vi "Run.vi"(8 "error in (no error)":errorcluster caption="entrée d'erreur (pas d'erreur)", 9 "Y":string[][](array[string]), 10 "X":string[][](array[string]), 11 "Pairwise_distances.lvclass":refnum<class "Pairwise_distances.lvclass">) -> (0 "error out":errorcluster caption="sortie d'erreur", 2 "Data":T1, 3 "Pairwise_distances.lvclass":refnum<class "Pairwise_distances.lvclass">)   [LabVIEW 2020, in "Pairwise_distances.lvclass"]
doc: "Returns : \n\n- D : array [n_samples_a, n_samples_a] or [n_samples_a, n_samples_b]\nA distance matrix D such that D_{i, j} is the distance between the ith and jth vectors of the given matrix X, if Y is None. If Y is not None, then D_{i, j} is the distance between the ith array from X and the jth array from Y."
uses:
  Pairwise_distances.lvclass
  Pairwise_distances.lvclass/Pairwise_distances.ctl
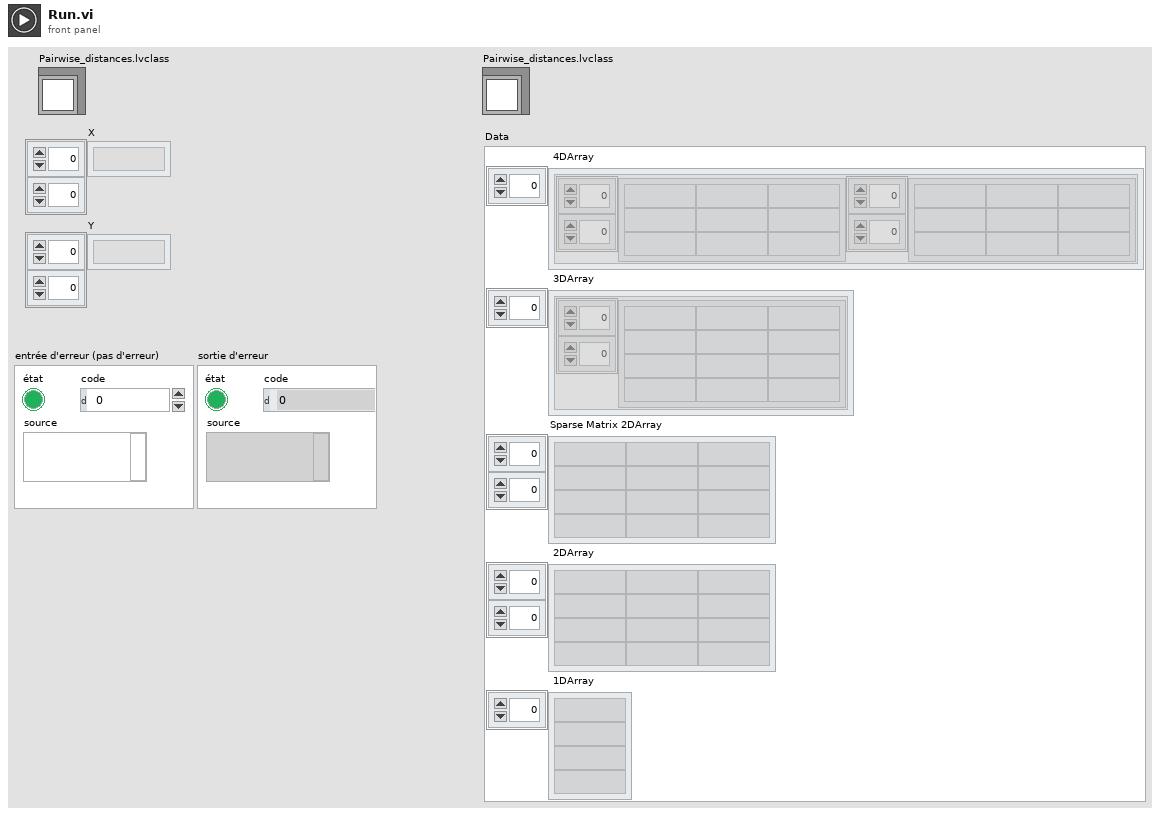
[diagram p1: front panel]
types:
  T1 = cluster{" 4DArray":cluster{"1":string[][], "2":string[][]}[], " 3DArray":cluster{"Tableau":string[][]}[], "Sparse Matrix 2DArray":string[][], " 2DArray":string[][], " 1DArray":string[]}
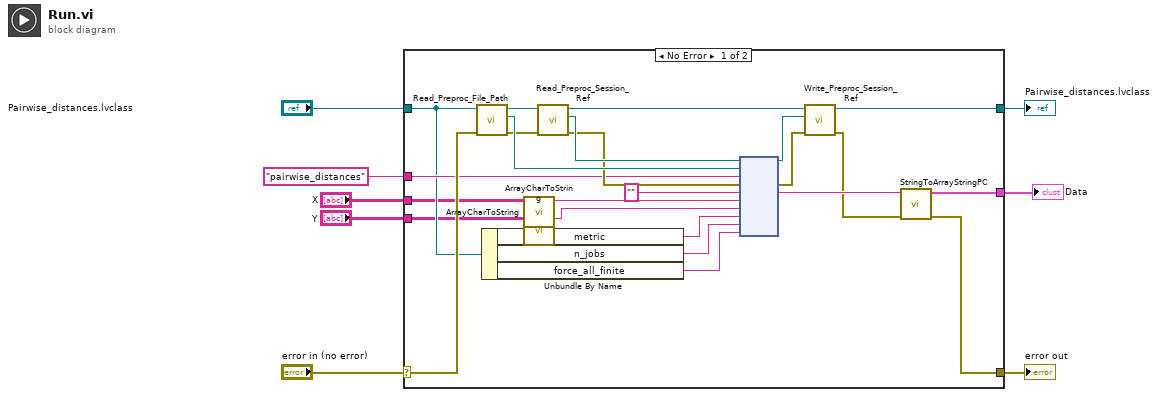
[diagram p0: block diagram]
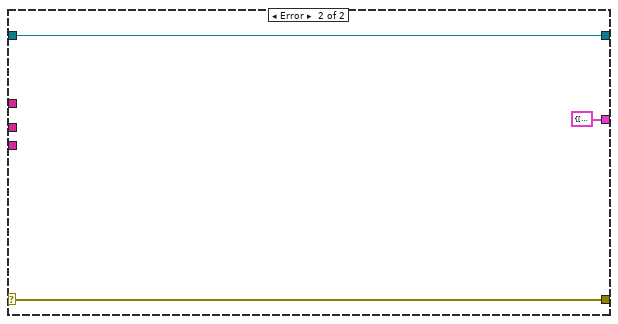
[diagram p2: hidden frame]
diagram:
  n1 = case shown="No Error" "error in (no error)" {
    selector: "error in (no error)" -> [w23 w35]
    tunnel: [w10 w35] -> w7
    tunnel: [w13 w34] -> w5
    tunnel: "Pairwise_distances.lvclass" -> [w21 w34]
    tunnel: "pairwise_distances" ("Fonction") -> [w22 _]
    tunnel: "X" -> [w17 _]
    tunnel: "Y" -> [w16 _]
    tunnel: [w9 T1 {" 4DArray"=[], " 3DArray"=[], "Sparse Matrix 2DArray"=[], " 2DArray"=[], " 1DArray"=[]} ("Data")] -> w1
    frame No Error {
      n2 = call-dynamic "Read_Preproc_File_Path.vi"("error in (no error)"=w23, "Python in"=w21) -> ("error out"=w27:errorcluster, "File_Path"=w30:path, "Python out"=w32:refnum<class "Pairwise_distances.lvclass">)  [unwired: 7 in]
      n3 = Unbundle By Name(w21) -> ("metric"=w20:string, "n_jobs"=w19:string, "force_all_finite"=w18:string)
      n4 = call "ArrayCharToString.vi"("TAB"=w17) -> ("Instruction"=w15:string)  [unwired: 10 in]
      n5 = call "ArrayCharToString.vi"("TAB"=w16) -> ("Instruction"=w14:string)  [unwired: 10 in]
      n6 = call-dynamic "Read_Preproc_Session_Ref.vi"("error in (no error)"=w27, "Python in"=w32) -> ("error out"=w28:errorcluster, "Session_ref"=w29:refnum<k35>, "Python out"=w31:refnum<class "Pairwise_distances.lvclass">)  [unwired: 7 in]
      n7 = node(w29, w30, w22, w28, "", w15, w14, w20, w19, w18) -> (w24:refnum<k35>, w26:errorcluster, w12:string)  [unwired: 5 in, 2 out]
      n8 = call-dynamic "Write_Preproc_Session_Ref.vi"("error in (no error)"=w26, "Session_ref"=w24, "Python in"=w31) -> ("error out"=w11:errorcluster, "Python out"=w13:refnum<class "Pairwise_distances.lvclass">)  [unwired: 7 in]
      n9 = call "StringToArrayStringPC.vi"("sortie d'erreur"=w11, "Return value"=w12) -> ("sortie d'erreur"=w10:errorcluster, "Data"=w9:T1)  [unwired: 8 in]
    }
    frame Error {
    }
  }
  "error out" <- w7
  "Pairwise_distances.lvclass" <- w5
  "Data" <- w1
